vi "HOST_feedbacktest_25beam_AAOptAOD6-27-23.vi"() -> ()   [LabVIEW 2020]
uses:
  <vilib>/userDefined/Silver/nirio_resource_slv.ctl
  Controls/Clock Select.ctl
  <vilib>/rvi/Analysis/control/PID/Typedef/niFpgaPID_ManualControl.ctl
  <vilib>/rvi/Analysis/control/PID/Typedef/niFpgaPID_PIDGains.ctl
  <vilib>/rvi/Analysis/control/PID/Typedef/niFpgaPID_OutputRange.ctl
  <vilib>/rvi/Analysis/control/PID/Typedef/niFpgaPID_SetpointWeightings.ctl
  <vilib>/rvi/Analysis/host/Butterworth/config/Butterworth Filter Order.ctl
  <vilib>/rvi/Analysis/host/Butterworth/config/Butterworth Filter Type.ctl
  <vilib>/FPGAPlugInAG/PXIe-7972R/niLvFpga_Open_PXIe-7972R.vi
  <vilib>/rvi/interface/common/dynamic/niFpgaDynamicAddResources.vi
  <vilib>/rvi/interface/common/niFpgaWaitOnOcc.vi
  <vilib>/Utility/error.llb/Error Cluster From Error Code.vi
  <vilib>/rvi/Analysis/host/Butterworth/config/BwScaledCoefficients.vi
  <vilib>/Utility/file.llb/Write Delimited Spreadsheet (string).vi
  <vilib>/rvi/errors/niLvFpgaAdjustHostInterfaceError.vi
  <instrlib>/_niInstr/Streaming/v1/Host/Public/Start Finite Stream.vi
  <instrlib>/_niInstr/Streaming/v1/Host/Public/Wait for Stream.vi
  <instrlib>/_niInstr/Streaming/v1/Host/Public/Start Continuous Stream.vi
  <vilib>/FPGAPlugInAG/Dynamic/niLvFpga_Close_Dynamic.vi
  <vilib>/rvi/interface/nirviOpenFPGA/nirviOpenFPGA.xnode
  FPGA Bitfiles/rfsignal_FPGATarget_feedbacktest25be_mYX3aSRDJfE.lvbitx
  <vilib>/rvi/interface/nirviMethod/nirviMethod.xnode
  <vilib>/rvi/Analysis/host/Butterworth/XNode/ButterworthCoefficients.xnode
  <vilib>/rvi/interface/nirviReadWriteControl/nirviReadWriteControl.xnode
  <vilib>/rvi/interface/nirviCloseFPGA/nirviCloseFPGA.xnode
  <vilib>/rvi/errors/niLvFpgaMergeErrorWithErrorCode.vi
  <instrlib>/_niInstr/Streaming/v1/Host/niInstr Streaming v1 Host.lvlib
  <vilib>/rvi/interface/Simulation/niFpgaSimulationCallBeginRW.vi
  NiFpgaLv.dll
  <vilib>/rvi/Analysis/host/Public/NI_FpgaMspHost.lvlib
  <vilib>/FPGAPlugInAG/Dynamic/niLvFpga_ConfigureFifo_Dynamic.vi
  <vilib>/FPGAPlugInAG/Dynamic/niLvFpga_StartFifo_Dynamic.vi
  <vilib>/FPGAPlugInAG/Dynamic/niLvFpga_WriteFifo_Dynamic.vi
panel:
  in  "Direction switch":bool
  in  "Step gain values":dbl
  in  "?":bool
  in  "Feedback out tester":bool
  in  "% of max CH 1":dbl=85.0
  in  "% of max CH 0":dbl=85.0
  in  "setpoint weighting":T1={"proportional weighting (1)"=1.0, "derivative weighting (0)"=0.0} {"derivative weighting (0)" min=0 max=1; "proportional weighting (1)" min=0 max=1}
  in  "output range":T2={"output high (Inf)"=inf, "output low (-Inf)"=-inf}
  in  "gains":T3 {"filter coefficient" min=0 max=1; "proportional gain" step=0.125}
  in  "manual control":T4
  in  "channel (0)":u8
  in  "reset? (F)":bool
  in  "PID selector":bool
  in  "write time ch0":bool
  in  "Record time for power sweep CH0":bool
  in  "Record time for power sweep CH1":bool
  in  "write time ch1":bool
  in  "save path for power calibration (dialog if empty)":path
  out "time check":u16=16
  in  "Cycles per step":u16=30
  in  "Gain Scan Endpoint (CH1)":dbl[](array[numeric])=[100.0, 100.0, 100.0, 100.0, 100.0, 100.0, 100.0, 100.0, 100.0, 100.0, 100.0, 100.0, 100.0, 100.0, 100.0, 100.0, 100.0, 100.0, 100.0, 100.0, 100.0, 100.0, 100.0, 100.0, 100.0, 100.0, 100.0, 100.0, 100.0, 100.0, 100.0, 100.0, 100.0, 100.0, 100.0, 100.0]
  in  "Gain Scan Endpoint (CH0)":dbl[](array[numeric])=[100.0, 100.0, 100.0, 100.0, 100.0, 100.0, 100.0, 100.0, 100.0, 100.0, 100.0, 100.0, 100.0, 100.0, 100.0, 100.0, 100.0, 100.0, 100.0, 100.0, 100.0, 100.0, 100.0, 100.0, 100.0, 100.0, 100.0, 100.0, 100.0, 100.0, 100.0, 100.0, 100.0, 100.0, 100.0, 100.0]
  in  "Scan End Setpoint (CH1)":dbl[](array[numeric])=[23.0, 24.0, 25.0, 26.0, 27.0, 28.0, 23.0, 24.0, 25.0, 26.0, 27.0, 28.0, 23.0, 24.0, 25.0, 26.0, 27.0, 28.0, 23.0, 24.0, 25.0, 26.0, 27.0, 28.0, 23.0, 24.0, 25.0, 26.0, 27.0, 28.0, 23.0, 24.0, 25.0, 26.0, 27.0, 28.0] format="%#_10f"
  in  "Scan CH1":bool
  in  "Scan CH0":bool
  in  "Fq Scan Endpoint (CH0)":dbl[](array[numeric])=[23.0, 23.0, 23.0, 23.0, 23.0, 23.0, 24.0, 24.0, 24.0, 24.0, 24.0, 24.0, 25.0, 25.0, 25.0, 25.0, 25.0, 25.0, 26.0, 26.0, 26.0, 26.0, 26.0, 26.0, 27.0, 27.0, 27.0, 27.0, 27.0, 27.0, 28.0, 28.0, 28.0, 28.0, 28.0, 28.0] format="%#_10f"
  in  "LP FF":dbl=5000.0 format="%#_13g"
  in  "Refresh Integral":bool
  in  "Setpoint Y 1":i16
  in  "Lower lim Y 1":fxp<+/-,16,16>=-300.0
  in  "Upper lim Y 1":fxp<+/-,16,16>=300.0
  in  "hp freq Y 1":dbl=1300.0
  in  "lp freq Y 1":dbl=1300.0
  out "AI 0 beam 1":cluster{"AI0":i16, "AI3":i16}(graph)={"AI0"=-30, "AI3"=-30}
  in  "Scaling (Y) 1":fxp<+,16,4>=1.0
  in  "D (Y) 1":fxp<+/-,16,16>
  in  "I (Y) 1":fxp<+/-,16,16>
  in  "P (Y) 1":fxp<+/-,16,16>
  in  "Amp mod on/off":bool[](array[boolean])=[FALSE, FALSE, FALSE, FALSE, FALSE, FALSE, FALSE, FALSE, FALSE]
  in  "Mod Amp (%)":fxp<+,16,1>[](array[numeric])=[1.0, 1.0, 1.0, 1.0, 1.0, 1.0, 1.0, 1.0, 1.0]
  in  "Mod Fq (Hz) 3":dbl[](array[numeric])=[1.0, 1.0, 1.0, 1.0, 1.0, 1.0, 1.0, 1.0, 1.0] format="%#5.5f"
  in  "Wave 2 mod on/off":bool[](array[boolean])=[FALSE, FALSE, FALSE, FALSE, FALSE, FALSE, FALSE, FALSE, FALSE]
  in  "Mod strength (Hz) 2":dbl[](array[numeric])=[100000.0, 100000.0, 100000.0, 100000.0, 100000.0, 100000.0, 100000.0, 100000.0, 100000.0] format="%#_6p"
  in  "Mod Fq (Hz) 2":dbl[](array[numeric])=[1.0, 1.0, 1.0, 1.0, 1.0, 1.0, 1.0, 1.0, 1.0] format="%#5.5f"
  in  "Wave 1 mod on/off":bool[](array[boolean])=[FALSE, FALSE, FALSE, FALSE, FALSE, FALSE, FALSE, FALSE, FALSE]
  in  "Mod strength (Hz)":dbl[](array[numeric])=[100000.0, 100000.0, 100000.0, 100000.0, 100000.0, 100000.0, 100000.0, 100000.0, 100000.0] format="%#_6p"
  in  "Mod Time (Hz)":dbl[](array[numeric])=[1.0, 1.0, 1.0, 1.0, 1.0, 1.0, 1.0, 1.0, 1.0] format="%#5.5p"
  in  "Gain Scan Step Size % (CH1)":dbl=1.0
  in  "Gain Scan Step Size % (CH0)":dbl=1.0
  in  "Fq Scan Step Size MHz (CH1)":dbl=0.1
  in  "Fq Scan Step Size MHz (CH0)":dbl=0.1
  in  "Input pass through\nmode":enum16{"Wire", "Accum", "Accum-edge"}(ring)
  in  "# of beams":i8=36
  in  "Wave Reader CH 1 (MHz)":dbl[](array[numeric])=[23.0, 24.0, 25.0, 26.0, 27.0, 28.0, 23.0, 24.0, 25.0, 26.0, 27.0, 28.0, 23.0, 24.0, 25.0, 26.0, 27.0, 28.0, 23.0, 24.0, 25.0, 26.0, 27.0, 28.0, 23.0, 24.0, 25.0, 26.0, 27.0, 28.0, 23.0, 24.0, 25.0, 26.0, 27.0, 28.0] format="%#_15f"
  in  "Gain CH 1 (%)":dbl[](array[numeric])=[100.0, 100.0, 100.0, 100.0, 100.0, 100.0, 100.0, 100.0, 100.0, 100.0, 100.0, 100.0, 100.0, 100.0, 100.0, 100.0, 100.0, 100.0, 100.0, 100.0, 100.0, 100.0, 100.0, 100.0, 100.0, 100.0, 100.0, 100.0, 100.0, 100.0, 100.0, 100.0, 100.0, 100.0, 100.0, 100.0]
  in  "Remove transition edges":i32=5
  in  "Time per beam in us":i32=20
  in  "stop":bool
  in  "Gain CH 0 (%)":dbl[](array[numeric])=[100.0, 100.0, 100.0, 100.0, 100.0, 100.0, 100.0, 100.0, 100.0, 100.0, 100.0, 100.0, 100.0, 100.0, 100.0, 100.0, 100.0, 100.0, 100.0, 100.0, 100.0, 100.0, 100.0, 100.0, 100.0, 100.0, 100.0, 100.0, 100.0, 100.0, 100.0, 100.0, 100.0, 100.0, 100.0, 100.0]
  in  "Wave Reader CH 0 (MHz)":dbl[](array[numeric])=[23.0, 23.0, 23.0, 23.0, 23.0, 23.0, 24.0, 24.0, 24.0, 24.0, 24.0, 24.0, 25.0, 25.0, 25.0, 25.0, 25.0, 25.0, 26.0, 26.0, 26.0, 26.0, 26.0, 26.0, 27.0, 27.0, 27.0, 27.0, 27.0, 27.0, 28.0, 28.0, 28.0, 28.0, 28.0, 28.0] format="%#_13f"
  in  "Magnitude Initialization Vpp":dbl[](array[numeric])=[1.0, 1.0] format="%0.2p"
  in  "Frequencies (Hz)":dbl[](array[numeric])=[10000.0, 10000.0] format="%5.0p"
  in  "Signal Type":T5(ring)
  in  "Sampling Info":cluster{"Fs":dbl, "#s":dbl}={"Fs"=163840000.0, "#s"=65536.0} {"Fs" format="%#_5p"}
  out "Error Out":errorcluster
  in  "Update Waveform":bool
  in  "Clock Select":T6 items=["Internal Clock", "Internal Clock w/ Ref via CLK/REF IN", "Internal Clock w/ Ref via Sync Clock", "External Clock via CLK/REF IN"]
  in  "Rate of External Sample Clock (MHz)":u16=100 min=60 max=100 step=1
  in  "RIO Resource":T7="RIO0"
  # "General Feedback Settings"
  # "Time cycle loop processing"
  # "Shared Feedback Controls"
  # "Don't change"
  # "Beam 1 Feedback Parameters"
  # "Waveform Initialization"
  # "Modulation disabled for now while testing FPGA code, too high compiling time for quick turn around"
  # "Controls the Output of the FPGA\nEach row corresponds to one beam created by the AOD\nCH 0 is Output 0 on the FPGA card and controls the () direction on the AOD; CH 1 is Output 1 on the FPGA card and controls the () direction on the AOD\n\nThe  set frequency is the output of the FPGA, this is then mixed with a 50MHz LO to be in the AOD's bandwidth of 75 +- 15MHz\n\nThe gain is the percentage of the 1Vpp initialized voltage to output. It is in percentage and goes from 0 - 100\n\nIt will play the first n rows of tones, \nwhere n is the \"# of beams\" value."
  # "DO NOT CHANGE"
  # "These allow you to smoothly ramp between frequencies or gain settings for each individual beam.\nThe channels scan independently, but it will simultaneously ramp every fq/gain in the channel to their desired point.\nThey should update to match the main control setting when scanning is not enabled."
  # "Ch 0 Wave Sin Modulation"
  # "Ch 1 Wave Sin Modulation"
  # "Amplitude Sin Modulation"
  # "Do not change these values while waiting for scan"
  # "Main control for the tones played on FPGA analog out 0\nSets the base, static frequency to play"
  # "Main control for the tones played on FPGA analog out 1\nSets the base, static frequency to play"
  # "Ch 0 Output Waveforms"
  # "Ch 1 Output Waveforms"
  # "Limits go as fractions of maxI16 (for testing purposes)\n1 means I16 positively saturated (dac output rails positive)\n-1 means I16 negatively saturated (dac output rails negative)\ndefined in PID subvi on the FPGA"
  # "Ch0"
  # "Ch1"
  # "Modulates the output frequencies of CH 0 in a sine wave pattern\n\nMod time: Sets how fast the modulation goes\n     (e.g. 1 Hz means it will go through a full cycle in 1 second)\n\nMod strength: Sets the amplitude of the modulation\n     (e.g. 100kHz means that the frequency will go between \n      set frequency + 100kHz and set frequency - 100kHz)"
  # "Modulates the output frequencies of CH 1 in a sine wave pattern\n\nMod time: Sets how fast the modulation goes\n     (e.g. 1 Hz means it will go through a full cycle in 1 second)\n\nMod strength: Sets the amplitude of the modulation\n     (e.g. 100kHz means that the frequency will go between \n      set frequency + 100kHz and set frequency - 100kHz)"
  # "Modulates the output amplitude of CH 0 in a sine wave pattern\n\nMod time: Sets how fast the modulation goes\n     (e.g. 1 Hz means it will go through a full cycle in 1 second)\n\nMod strength: Sets the amplitude of the modulation\n     (e.g. 5% means that the amplitude will go between \n      set amp + 5%  and set amp  - 5%)"
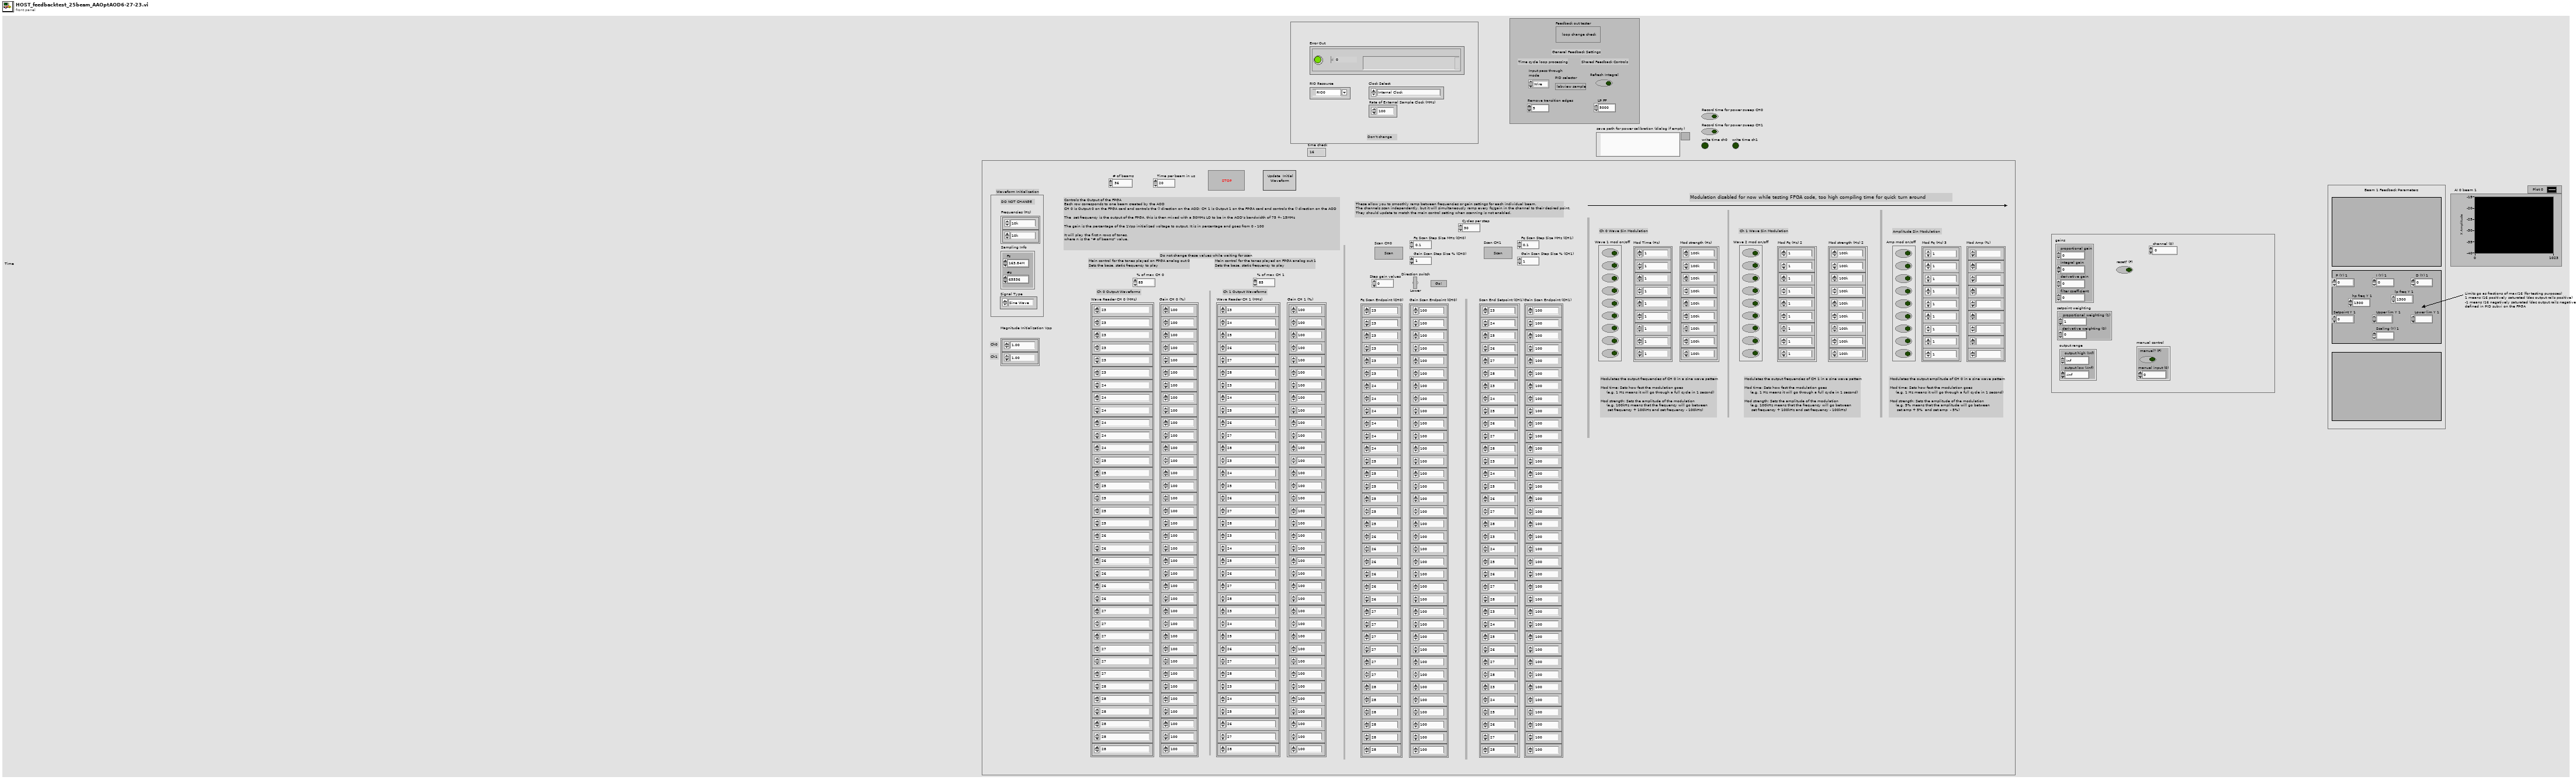
[diagram p1: front panel]
types:
  T1 = typedef "niFpgaPID_SetpointWeightings.ctl" = cluster{"proportional weighting (1)":sgl, "derivative weighting (0)":sgl}
  T2 = typedef "niFpgaPID_OutputRange.ctl" = cluster{"output high (Inf)":sgl, "output low (-Inf)":sgl}
  T3 = typedef "niFpgaPID_PIDGains.ctl" = cluster{"proportional gain":sgl, "integral gain":sgl, "derivative gain":sgl, "filter coefficient":sgl}
  T4 = typedef "niFpgaPID_ManualControl.ctl" = cluster{"manual? (F)":bool, "manual input (0)":sgl}
  T5 = enum16{"Sine Wave", "Triangle Wave", "Square Wave", "Sawtooth Wave"}
  T6 = typedef "Clock Select.ctl" = u16
  T7 = typedef "nirio_resource_slv.ctl" = tag
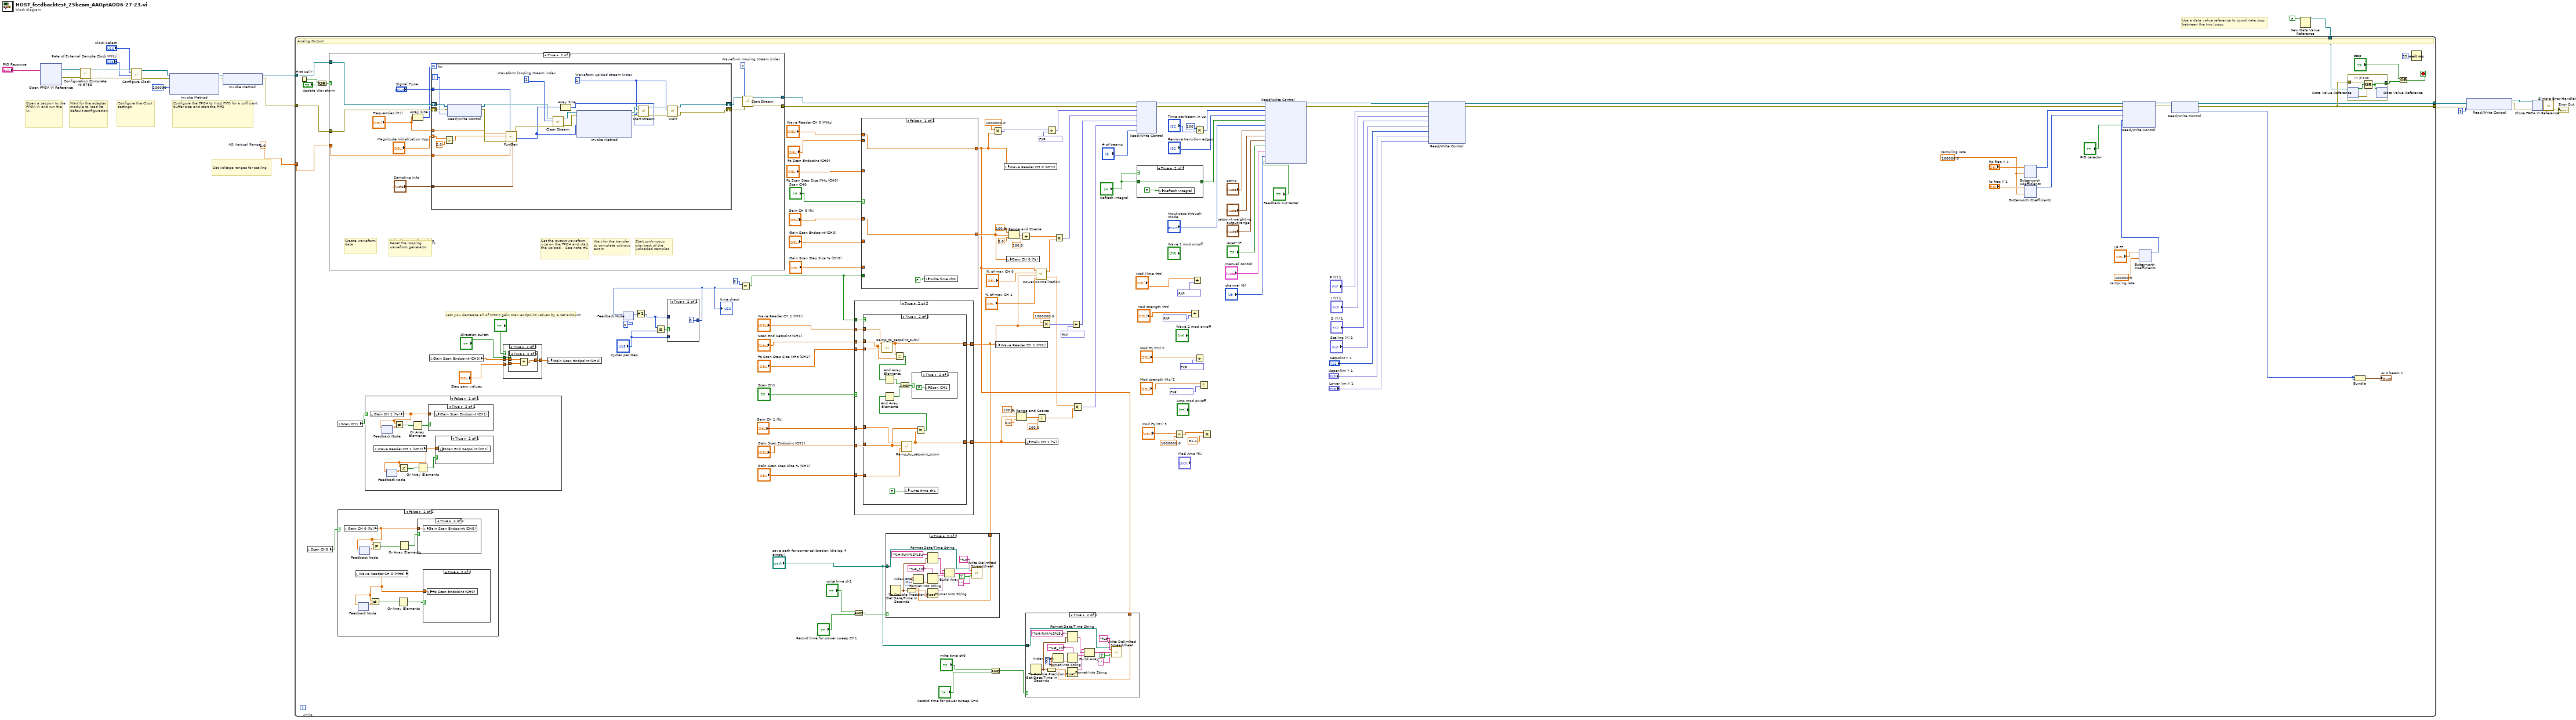
[diagram p0: block diagram]
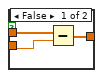
[diagram p3: hidden frame]
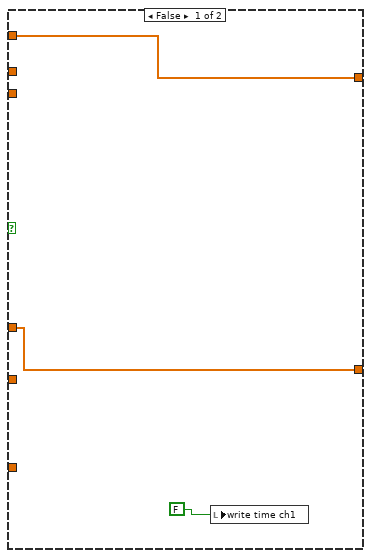
[diagram p6: hidden frame]
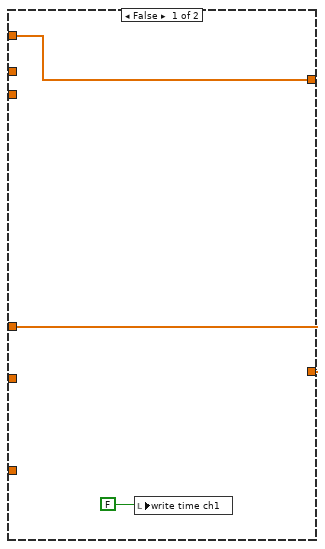
[diagram p7: hidden frame]
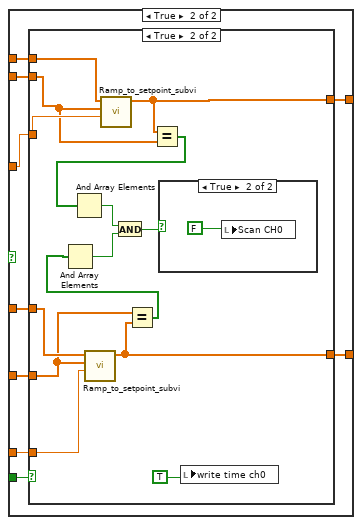
[diagram p9: hidden frame]
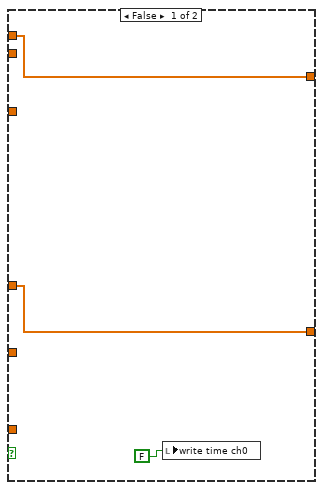
[diagram p10: hidden frame]
diagram:
  w12 = 1.0  # AO Vertical Range
  # "Use a data value reference to coordinate stop between the two loops"
  # "Set Voltage ranges for scaling"
  # "Configure the Clock settings"
  # "Configure the FPGA to Host FIFO for a sufficient buffer size and start the FIFO"
  # "Wait for the adapter module to load its default configuration."
  # "Open a session to the FPGA VI and run the VI."
  n1 = xnode "Open FPGA VI Reference"("resource name"="RIO Resource") -> ("FPGA VI Reference Out"=w10:refnum<k20>, "error out"=w9:errorcluster)  [unwired: 1 in]
  n2 = call "Configuration Complete NI 5783.vi"("error in"=w9, "FPGA VI Reference In"=w10) -> ("error out"=w20:errorcluster, "FPGA VI Reference Out"=w21:refnum<k20>)  [unwired: 7 in, 1 out]
  n3 = call "Configure Clock.vi"("error in (no error)"=w20, "Rate of External Sample Clock (MHz)"="Rate of External Sample Clock (MHz)", "Clock Select"="Clock Select", "FPGA VI Reference In"=w21) -> ("error out"=w18:errorcluster, "FPGA VI Reference Out"=w19:refnum<k20>)  [unwired: 3 in, 3 out]
  n4 = xnode "Invoke Method"("FPGA VI Reference In"=w19, "error in"=w18, "Requested Depth"=u32 100000) -> ("FPGA VI Reference Out"=w24:refnum<k20>, "error out"=w23:errorcluster)  [unwired: 1 out]
  n5 = xnode "Invoke Method"("FPGA VI Reference In"=w24, "error in"=w23) -> ("FPGA VI Reference Out"=w3:refnum<k20>, "error out"=w2:errorcluster)
  n6 = New Data Value Reference(data value=FALSE ("Stopped")) -> (data value reference=w1:refnum<data-value>)  [unwired: 1 in, 1 out]
  n7 = while {
    tunnel: w2 -> [w150]
    tunnel: [w117] -> w8
    tunnel: w3 -> [w156]
    tunnel: [w102] -> w7
    tunnel: w1 -> [w151]
    tunnel: w12 -> [w149]
    stop <- w146 stop-if-true
    w96 = 100000.0  # sampling rate
    w103 = 100000.0  # sampling rate
    # "Lets you decrease all of CH0's gain scan endpoint values by a set amount"
    # "Analog Output"
    n8 = First Call?() -> (First Call?: T/F=w152:bool)
    n9 = local read "Scan CH0"() -> (w71:bool)
    n10 = Or(x=w152, y="Update Waveform") -> (x .or. y?=w153:bool)
    n11 = case shown="True" w153 {
      tunnel: [w309 w322] -> w148
      tunnel: [w308 w321] -> w147
      tunnel: w156 -> [w309 w319]
      tunnel: w150 -> [w308 w318]
      tunnel: w149 -> [_ w320]
      frame False {
      }
      frame True {
        w317 = 2  # Waveform looping stream index
        # "Loop over the waveforms to combine"
        # "Reset the looping waveform generator"
        # "Start continuous playback of the uploaded samples"
        # "Wait for the transfer to complete without errors"
        # "Set the output waveform size on the FPGA and start the upload.   See note #1"
        # "Write the waveform data to the FPGA for generation"
        # "Create waveform data"
        n12 = Array Size(array="Frequencies (Hz)") -> (size(s)=w312:i32)
        n13 = for {
          N: w312 -> [_]
          tunnel: w320 -> [w337]
          shift-right: [w331] -> w316
          shift-left: w319 -> [w336]
          shift-right: [w330] -> w315
          shift-left: w318 -> [w334]
          tunnel: "Frequencies (Hz)" -> [w329] mode=indexing
          tunnel: "Magnitude Initialization Vpp" -> [w325] mode=indexing
          tunnel: "Sampling Info" -> [w328]
          tunnel: "Signal Type" -> [w327]
          i -> [w326]
          w338 = 2  # Waveform looping stream index
          w343 = 1  # Waveform upload stream index
          n14 = Divide(x=w325, y=2.0) -> (x/y=w324:dbl)
          n15 = xnode "Read/Write Control"("FPGA VI Reference In"=w336, "error in"=w334, "Upload selector"=w326) -> ("FPGA VI Reference Out"=w335:refnum<k20>, "error out"=w333:errorcluster)
          n16 = call "FunGen.vi"("sampling info"=w328, "range (Vpp)"=w337, "signal type"=w327, "error in (no error)"=w333, "amplitude"=w324, "frequency"=w329) -> ("error out"=w339:errorcluster, "Waveform Data"=w332:i16[])  [unwired: 2 in, 2 out]
          n17 = call <instrlib>:"Clear Stream.vi"("error in (no error)"=w339, "stream index"=w338, "refnum in"=w335) -> ("error out"=w341:errorcluster, "refnum out"=w342:refnum<k20>)  [unwired: 7 in]
          n18 = Array Size(array=w332) -> (size(s)=w340:i32)
          n19 = xnode "Invoke Method"("FPGA VI Reference In"=w342, "error in"=w341, "Data"=w332) -> ("FPGA VI Reference Out"=w347:refnum<k20>, "error out"=w346:errorcluster)  [unwired: 1 in, 1 out]
          n20 = call-poly <instrlib>:"Start Stream.vi"("error in (no error)"=w346, "num samples"=w340, "stream index"=w343, "refnum in"=w347) -> ("error out"=w344:errorcluster, "refnum out"=w345:refnum<k20>)  [unwired: 6 in]
          n21 = call-poly <instrlib>:"Wait.vi"("error in (no error)"=w344, "stream index"=w343, "refnum in"=w345) -> ("error out"=w330:errorcluster, "refnum out"=w331:refnum<k20>)  [unwired: 5 in, 2 out]
        }
        n22 = call-poly <instrlib>:"Start Stream.vi"("error in (no error)"=w315, "stream index"=w317, "refnum in"=w316) -> ("error out"=w321:errorcluster, "refnum out"=w322:refnum<k20>)  [unwired: 7 in]
      }
    }
    n23 = local read "Scan CH1"() -> (w72:bool)
    n24 = case shown="False" w71 {
      frame False {
        n25 = local read "Gain CH 0 (%)"() -> (w260:dbl[])
        n26 = local read "Wave Reader CH 0 (MHz)"() -> (w267:dbl[])
        n27 = feedback-in #1(w267) -> ()
        n28 = feedback #1() -> (w266:dbl[])  [unwired: 1 in]
        n29 = feedback #2() -> (w263:dbl[])  [unwired: 1 in]
        n30 = feedback-in #2(w260) -> ()
        n31 = Not Equal?(x=w267, y=w266) -> (x != y?=w265:bool[])
        n32 = Not Equal?(x=w260, y=w263) -> (x != y?=w262:bool[])
        n33 = Or Array Elements(Boolean array=w265) -> (logical OR=w264:bool)
        n34 = Or Array Elements(Boolean array=w262) -> (logical OR=w261:bool)
        n35 = case shown="True" w261 {
          tunnel: w260 -> [_ w268]
          frame False {
          }
          frame True {
            n36 = local write "Gain Scan Endpoint (CH0)"(w268) -> ()
          }
        }
        n37 = case shown="True" w264 {
          tunnel: w267 -> [_ w269]
          frame False {
          }
          frame True {
            n38 = local write "Fq Scan Endpoint (CH0)"(w269) -> ()
          }
        }
      }
      frame True {
      }
    }
    n39 = case shown="False" w72 {
      frame False {
        n40 = local read "Gain CH 1 (%)"() -> (w270:dbl[])
        n41 = local read "Wave Reader CH 1 (MHz)"() -> (w274:dbl[])
        n42 = feedback #3() -> (w273:dbl[])  [unwired: 1 in]
        n43 = feedback-in #3(w270) -> ()
        n44 = feedback #4() -> (w277:dbl[])  [unwired: 1 in]
        n45 = feedback-in #4(w274) -> ()
        n46 = Not Equal?(x=w270, y=w273) -> (x != y?=w272:bool[])
        n47 = Not Equal?(x=w274, y=w277) -> (x != y?=w276:bool[])
        n48 = Or Array Elements(Boolean array=w272) -> (logical OR=w271:bool)
        n49 = Or Array Elements(Boolean array=w276) -> (logical OR=w275:bool)
        n50 = case shown="True" w271 {
          tunnel: w270 -> [_ w278]
          frame False {
          }
          frame True {
            n51 = local write "Gain Scan Endpoint (CH1)"(w278) -> ()
          }
        }
        n52 = case shown="True" w275 {
          tunnel: w274 -> [_ w279]
          frame False {
          }
          frame True {
            n53 = local write "Scan End Setpoint (CH1)"(w279) -> ()
          }
        }
      }
      frame True {
      }
    }
    n54 = local read "Gain Scan Endpoint (CH0)"() -> (w26:dbl[])
    n55 = case shown="True" "?" {
      tunnel: w26 -> [w157 w160]
      tunnel: [w157 w161] -> w27
      tunnel: "Step gain values" -> [_ w159]
      tunnel: "Direction switch" -> [_ w158]
      frame False {
      }
      frame True {
        n56 = case shown="True" w158 {
          tunnel: [w164 w166] -> w161
          tunnel: w160 -> [w163 w165]
          tunnel: w159 -> [w162 w167]
          frame False {
            n57 = Subtract(x=w163, y=w162) -> (x-y=w164:dbl[])
          }
          frame True {
            n58 = Add(x=w165, y=w167) -> (x+y=w166:dbl[])
          }
        }
      }
    }
    n59 = local write "Gain Scan Endpoint (CH0)"(w27) -> ()
    n60 = feedback #5(u16 0) -> (w67:u16)
    n61 = Increment(x=w67) -> (x+1=w65:u16)
    n62 = Greater Or Equal?(x=w65, y="Cycles per step") -> (x >= y?=w66:bool)
    n63 = case shown="True" w66 {
      tunnel: w65 -> [w258 _]
      tunnel: "Cycles per step" -> [_ _]
      tunnel: [w258 u16 0] -> w60
      frame False {
      }
      frame True {
      }
    }
    "time check" <- w60
    n64 = feedback-in #5(w60) -> ()
    n65 = Equal?(x=u16 0, y=w60) -> (x = y?=w61:bool)
    n66 = And(x="write time ch1", y="Record time for power sweep CH1") -> (x .and. y?=w59:bool)
    n67 = case shown="True" "Scan CH1" {
      tunnel: "Fq Scan Step Size MHz (CH1)" -> [_ w209]
      tunnel: [w200 w208] -> w36
      tunnel: "Wave Reader CH 1 (MHz)" -> [w200 w207]
      tunnel: "Scan End Setpoint (CH1)" -> [_ w206]
      tunnel: "Gain Scan Step Size % (CH1)" -> [_ w205]
      tunnel: "Gain CH 1 (%)" -> [w199 w204]
      tunnel: "Gain Scan Endpoint (CH1)" -> [_ w203]
      tunnel: [w199 w202] -> w73
      tunnel: w61 -> [_ w201]
      frame False {
        n68 = local write "write time ch1"(FALSE) -> ()
      }
      frame True {
        n69 = case shown="True" w201 {
          tunnel: w207 -> [w212 w226]
          tunnel: w206 -> [_ w224]
          tunnel: w209 -> [_ w225]
          tunnel: [w212 w223] -> w208
          tunnel: w204 -> [w211 w221]
          tunnel: w203 -> [_ w220]
          tunnel: w205 -> [_ w219]
          tunnel: [w211 w214] -> w202
          frame False {
            n70 = local write "write time ch1"(FALSE) -> ()
          }
          frame True {
            n71 = call "Ramp_to_setpoint_subvi.vi"("Numeric"=w225, "Scan to Fq (CH0)"=w224, "Wave Reader CH 0 (Y)"=w226) -> ("Array"=w223:dbl[])  [unwired: 8 in]
            n72 = Equal?(x=w223, y=w224) -> (x = y?=w222:bool[])
            n73 = And Array Elements(Boolean array=w222) -> (logical AND=w216:bool)
            n74 = call "Ramp_to_setpoint_subvi.vi"("Numeric"=w219, "Scan to Fq (CH0)"=w220, "Wave Reader CH 0 (Y)"=w221) -> ("Array"=w214:dbl[])  [unwired: 8 in]
            n75 = local write "write time ch1"(TRUE) -> ()
            n76 = Equal?(x=w220, y=w214) -> (x = y?=w215:bool[])
            n77 = And Array Elements(Boolean array=w215) -> (logical AND=w217:bool)
            n78 = And(x=w216, y=w217) -> (x .and. y?=w218:bool)
            n79 = case shown="True" w218 {
              frame False {
              }
              frame True {
                n80 = local write "Scan CH1"(FALSE) -> ()
              }
            }
          }
        }
      }
    }
    n81 = case shown="False" "Scan CH0" {
      tunnel: "Fq Scan Step Size MHz (CH0)" -> [_ w239]
      tunnel: "Wave Reader CH 0 (MHz)" -> [w230 w238]
      tunnel: "Fq Scan Endpoint (CH0)" -> [_ w237]
      tunnel: [w230 w236] -> w37
      tunnel: "Gain CH 0 (%)" -> [w229 w235]
      tunnel: "Gain Scan Endpoint (CH0)" -> [_ w234]
      tunnel: [w229 w233] -> w81
      tunnel: "Gain Scan Step Size % (CH0)" -> [_ w232]
      tunnel: w61 -> [_ w231]
      frame False {
        n82 = local write "write time ch0"(FALSE) -> ()
      }
      frame True {
        n83 = case shown="True" w231 {
          tunnel: w238 -> [w242 w256]
          tunnel: w237 -> [_ w254]
          tunnel: w239 -> [_ w255]
          tunnel: [w242 w253] -> w236
          tunnel: w235 -> [w241 w251]
          tunnel: w234 -> [_ w248]
          tunnel: w232 -> [_ w250]
          tunnel: [w241 w249] -> w233
          frame False {
            n84 = local write "write time ch0"(FALSE) -> ()
          }
          frame True {
            n85 = call "Ramp_to_setpoint_subvi.vi"("Numeric"=w250, "Scan to Fq (CH0)"=w248, "Wave Reader CH 0 (Y)"=w251) -> ("Array"=w249:dbl[])  [unwired: 8 in]
            n86 = call "Ramp_to_setpoint_subvi.vi"("Numeric"=w255, "Scan to Fq (CH0)"=w254, "Wave Reader CH 0 (Y)"=w256) -> ("Array"=w253:dbl[])  [unwired: 8 in]
            n87 = Equal?(x=w248, y=w249) -> (x = y?=w247:bool[])
            n88 = And Array Elements(Boolean array=w247) -> (logical AND=w244:bool)
            n89 = Equal?(x=w253, y=w254) -> (x = y?=w252:bool[])
            n90 = And Array Elements(Boolean array=w252) -> (logical AND=w245:bool)
            n91 = And(x=w245, y=w244) -> (x .and. y?=w246:bool)
            n92 = case shown="True" w246 {
              frame False {
              }
              frame True {
                n93 = local write "Scan CH0"(FALSE) -> ()
              }
            }
            n94 = local write "write time ch0"(TRUE) -> ()
          }
        }
      }
    }
    n95 = case shown="True" w59 {
      tunnel: w36 -> [_ w190]
      tunnel: "save path for power calibration (dialog if empty)" -> [_ w183]
      frame False {
      }
      frame True {
        n96 = Get Date/Time In Seconds() -> (seconds since 1Jan1904=w186:timestamp)
        n97 = To Double Precision Float(number=w186) -> (double precision float=w185:dbl)
        n98 = Index Array(array=w190, index=0) -> (element=w188:dbl)
        n99 = Format Date/Time String(time format string (%c)="%H:%M:%S%3u", seconds (now)=w186) -> (date/time string=w193:string)  [unwired: 1 in]
        n100 = Format Into String(format string="%#_10f", w188) -> (resulting string=w192:string)  [unwired: 2 in, 1 out]
        n101 = Format Into String(w185) -> (resulting string=w184:string)  [unwired: 3 in, 1 out]
        n102 = Build Array(w184, w193, w192) -> (w187:string[])
        n103 = call-poly <vilib>:"Write Delimited Spreadsheet.vi"("file path (dialog if empty)"=w183, "format (%s)"="%s" ("format (%.3f)"), "1D data"=w187, "append to file? (new file:F)"=TRUE, "delimiter (\\t)"="," ("delimiter (\\t)")) -> ()  [unwired: 9 in, 2 out]
      }
    }
    n104 = And(x="write time ch0", y="Record time for power sweep CH0") -> (x .and. y?=w55:bool)
    n105 = Multiply(x=1000000.0, y=w37) -> (x*y=w93:fxp<+/-,64,32>[])
    n106 = local write "Wave Reader CH 1 (MHz)"(w36) -> ()
    n107 = local write "Wave Reader CH 0 (MHz)"(w37) -> ()
    n108 = local write "Gain CH 0 (%)"(w81) -> ()
    n109 = In Range and Coerce(upper limit=100.0, x=w81, lower limit=0.0) -> (coerced(x)=w84:dbl[])  [unwired: 1 out]
    n110 = In Range and Coerce(upper limit=100.0, x=w73, lower limit=0.0) -> (coerced(x)=w79:dbl[])  [unwired: 1 out]
    n111 = Divide(x=w84, y=100.0) -> (x/y=w41:dbl[])
    n112 = local write "Gain CH 1 (%)"(w73) -> ()
    n113 = case shown="True" w55 {
      tunnel: w37 -> [_ w175]
      tunnel: "save path for power calibration (dialog if empty)" -> [_ w168]
      frame False {
      }
      frame True {
        n114 = Get Date/Time In Seconds() -> (seconds since 1Jan1904=w171:timestamp)
        n115 = To Double Precision Float(number=w171) -> (double precision float=w170:dbl)
        n116 = Index Array(array=w175, index=0) -> (element=w173:dbl)
        n117 = Format Date/Time String(time format string (%c)="%H:%M:%S%3u", seconds (now)=w171) -> (date/time string=w178:string)  [unwired: 1 in]
        n118 = Format Into String(format string="%#_10f", w173) -> (resulting string=w177:string)  [unwired: 2 in, 1 out]
        n119 = Format Into String(w170) -> (resulting string=w169:string)  [unwired: 3 in, 1 out]
        n120 = Build Array(w169, w178, w177) -> (w172:string[])
        n121 = call-poly <vilib>:"Write Delimited Spreadsheet.vi"("file path (dialog if empty)"=w168, "format (%s)"="%s" ("format (%.3f)"), "1D data"=w172, "append to file? (new file:F)"=TRUE, "delimiter (\\t)"="," ("delimiter (\\t)")) -> ()  [unwired: 9 in, 2 out]
      }
    }
    n122 = call "Power normalization.vi"("% of max CH 1"="% of max CH 1", "CH 1 frequency"=w36, "% of max CH 0"="% of max CH 0", "CH 0 frequency"=w37) -> ("Normalized CH1"=w33:dbl[], "Normalized CH 0"=w38:dbl[])
    n123 = Divide(x=w79, y=100.0) -> (x/y=w34:dbl[])
    n124 = Multiply(x=1000000.0, y=w36) -> (x*y=w90:fxp<+/-,64,32>[])
    n125 = Divide(x=w93, y=fxp<+,32,16> 6103.515625) -> (x/y=w51:fxp<+,33,16>[])
    n126 = Multiply(x=w41, y=w38) -> (x*y=w42:fxp<+,32,4>[])
    n127 = Divide(x=w90, y=fxp<+,32,16> 6103.515625) -> (x/y=w50:fxp<+,33,16>[])
    n128 = Multiply(x=w33, y=w34) -> (x*y=w35:fxp<+,32,4>[])
    n129 = case shown="True" "Refresh Integral" {
      tunnel: [w280 w281] -> w95
      tunnel: "Refresh Integral" -> [w280 w281]
      frame False {
      }
      frame True {
        n130 = local write "Refresh Integral"(FALSE) -> ()
      }
    }
    n131 = xnode "Read/Write Control"("FPGA VI Reference In"=w148, "error in"=w147, "Wave 1"=w51, "Amp 1"=w42, "Wave 2"=w50, "Amp 2"=w35, "Size"="# of beams") -> ("FPGA VI Reference Out"=w142:refnum<k20>, "error out"=w141:errorcluster)
    n132 = Divide(x="Mod Fq (Hz) 3", y=1000000.0) -> (x/y=w127:dbl[])
    n133 = Divide(x="Mod strength (Hz)", y=fxp<+,32,16> 6103.515625) -> ()  [unwired: 1 out]
    n134 = Divide(x="Mod Time (Hz)", y=fxp<+,32,16> 6103.515625) -> ()  [unwired: 1 out]
    n135 = Divide(x="Mod Fq (Hz) 2", y=fxp<+,32,16> 6103.515625) -> ()  [unwired: 1 out]
    n136 = Multiply(x=100, y="Time per beam in us") -> (x*y=w138:i32)
    n137 = Divide(x="Mod strength (Hz) 2", y=fxp<+,32,16> 6103.515625) -> ()  [unwired: 1 out]
    n138 = Multiply(x=w127, y=51.2) -> ()  [unwired: 1 out]
    n139 = xnode "Read/Write Control"("FPGA VI Reference In"=w142, "error in"=w141, "Timeshare"=w138, "Edge size"="Remove transition edges", "Integral reset"=w95, "Pass selector"="Input pass through\nmode", "gains"="gains", "setpoint weighting"="setpoint weighting", "output range"="output range", "reset? (F)"="reset? (F)", "manual control"="manual control", "channel (0)"="channel (0)", "Feedback out tester"="Feedback out tester") -> ("FPGA VI Reference Out"=w131:refnum<k20>, "error out"=w130:errorcluster)
    n140 = xnode "Read/Write Control"("FPGA VI Reference In"=w131, "error in"=w130, "Py gain 1"="P (Y) 1", "Iy gain 1"="I (Y) 1", "Dy gain 1"="D (Y) 1", "Feedback scaling"="Scaling (Y) 1", "Y DC offset 1"="Setpoint Y 1", "Y up lim 1"="Upper lim Y 1", "Y low lim 1"="Lower lim Y 1") -> ("FPGA VI Reference Out"=w108:refnum<k20>, "error out"=w107:errorcluster)
    n141 = xnode "Butterworth Coefficients"("cutoff frequency (Hz)"="hp freq Y 1", "sample rate (S/s)"=w103) -> ("scaled coefficients"=w100:i32[])  [unwired: 1 in, 1 out]
    n142 = xnode "Butterworth Coefficients"("cutoff frequency (Hz)"="lp freq Y 1", "sample rate (S/s)"=w103) -> ("scaled coefficients"=w99:i32[])  [unwired: 1 in, 1 out]
    n143 = xnode "Butterworth Coefficients"("cutoff frequency (Hz)"="LP FF", "sample rate (S/s)"=w96) -> ("scaled coefficients"=w52:i32[])  [unwired: 1 in, 1 out]
    n144 = xnode "Read/Write Control"("FPGA VI Reference In"=w108, "error in"=w107, "Y hp coef 1"=w100, "Y lp coef 1"=w99, "Final filter coef"=w52, "PID selector"="PID selector") -> ("FPGA VI Reference Out"=w101:refnum<k20>, "error out"=w98:errorcluster)
    n145 = xnode "Read/Write Control"("FPGA VI Reference In"=w101, "error in"=w98) -> ("FPGA VI Reference Out"=w102:refnum<k20>, "error out"=w117:errorcluster, "AI 0 input 1"=w104:i16)
    n146 = in-place {
      in-place-border: [w305] -> w145
      in-place-border: w117 -> [w307]
      n147 = in-place-dvr #6(w151) -> (w306:bool, w304:errorcluster)
      n148 = Compound Arithmetic op=OR(w307, w306, w304) -> (w305:bool)
      n149 = in-place-dvr #6(w305) -> ()  [unwired: 2 out]
    }
    n150 = Bundle("AI 0 input 1"=w104, "AI 0 input 1"=w104) -> (→"AI 0 beam 1":cluster{"AI 0 input 1":i16, "AI 0 input 1":i16})  [unwired: 1 in]
    n151 = Or(x="stop", y=w145) -> (x .or. y?=w146:bool)
    n152 = Wait (ms)(milliseconds to wait=u32 33) -> ()  [unwired: 1 out]
  }
  n153 = xnode "Read/Write Control"("FPGA VI Reference In"=w7, "error in"=w8, "stream.request state 2"=3) -> ("FPGA VI Reference Out"=w4:refnum<k20>, "error out"=w6:errorcluster)
  n154 = xnode "Close FPGA VI Reference"("FPGA VI Reference In"=w4, "error in"=w6) -> ("error out"=w15:errorcluster)
  n155 = call <vilib>:"Simple Error Handler.vi"("error in (no error)"=w15) -> ("error out"=→"Error Out":errorcluster)  [unwired: 4 in, 4 out]
